vi "Write Config File Handle.vi"(10 "Session Handle":T1, 11 "User Interface in":refnum<class "User Interface.lvclass">) -> (3 "User Interface out":refnum<class "User Interface.lvclass">)   [LabVIEW 2016, in "_User Interface.lvlib" / "User Interface.lvclass"]
uses:
  User Interface.lvclass
  Configurations.lvclass
  Session Handle.ctl
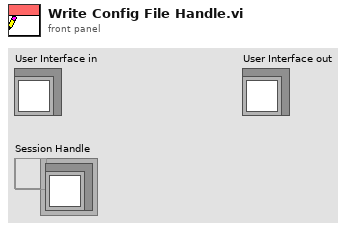
[diagram p1: front panel]
types:
  T1 = typedef "Configurations.lvlib/Configurations.lvclass/Session Handle.ctl" = refnum<data-value>
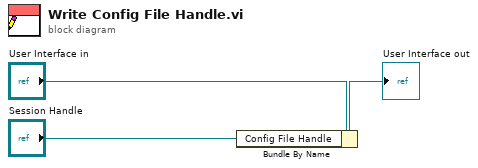
[diagram p0: block diagram]
diagram:
  n1 = Bundle By Name(cluster="User Interface in", "Config File Handle"="Session Handle") -> (→"User Interface out":refnum<class "User Interface.lvclass">)
